vi "svfa_Modify Enhanced Spectrum Info (Dual).vi"(0 "spectrum info X":T3={"channel name"="", "description"="", "x-axis units"=0, "spectral info"={"spectrum type"=enum."Power [Magnitude^2]", "linear/dB"=enum."linear", "window"=0, "window size"=0, "FFT size"=0}, "engineering units"=0, "custom label"="", "dB reference [EU]"=0.0, "peak units"=enum."rms", "weighting filter"=0, "spectral density?"=FALSE, "unit label"="", "spectrum skewed?"=FALSE, "complimentary spectrum units"=enum."none"} {"x-axis units" items=["Time (s)"=0, "Frequency-CB (Hz)"=1, "Frequency-CPB (Hz)"=1248, "Frequency-Arbitrary (Hz)"=2357, "Quefrency (s)"=2, "Revolutions (rev)"=3, "Order"=4, "Speed (RPM)"=11, "Speed (rad/s)"=21, "Index"=65535]; "weighting filter" items=["Linear", "A-weighting", "B-weighting", "C-weighting", "ITU-R 468-4", "Dolby", "CCITT", "C-message", "Wb", "Wc", "Wd", "We", "Wf", "Wh", "Wj", "Wk", "Wm", "AES17 20 kHz lowpass", "AES17 40 kHz lowpass", "AES17 20 kHz highpass", "AES17 40 kHz highpass"]; "dB reference [EU]" format="%.2f"; "engineering units" items=["custom..."=0, "V"=1, "A"=21, "C"=30, "pC"=31, "s"=32, "-"=29, "Pa"=2, "N"=20, "g"=3, "m/s^2"=4, "m/s"=5, "m"=6, "mm/s"=12, "mm"=13, "micron/s"=14, "micron"=15, "in/s^2"=7, "in/s"=8, "in"=9, "mil/s"=10, "mil"=11, "rad/s^2"=16, "rad/s"=17, "rad"=18, "deg/s^2"=26, "deg/s"=27, "deg"=28, "RPM"=22, "cycle/s^2"=23, "Hz"=24, "cycle"=25, "strain"=19]; "spectral info"."window" items=["None "=0, "Hanning"=1, "Hamming"=2, "Blackman-Harris"=3, "Exact Blackman"=4, "Blackman"=5, "Flat Top"=6, "4 Term B-Harris "=7, "7 Term B-Harris"=8, "Low Sidelobe"=9, "Force - Exponential"=10, "Gaussian"=62]}, 1 "processing control":T1(ring), 5 "spectrum info Y":T3={"channel name"="", "description"="", "x-axis units"=0, "spectral info"={"spectrum type"=enum."Power [Magnitude^2]", "linear/dB"=enum."linear", "window"=0, "window size"=0, "FFT size"=0}, "engineering units"=0, "custom label"="", "dB reference [EU]"=0.0, "peak units"=enum."rms", "weighting filter"=0, "spectral density?"=FALSE, "unit label"="", "spectrum skewed?"=FALSE, "complimentary spectrum units"=enum."none"} {"x-axis units" items=["Time (s)"=0, "Frequency-CB (Hz)"=1, "Frequency-CPB (Hz)"=1248, "Frequency-Arbitrary (Hz)"=2357, "Quefrency (s)"=2, "Revolutions (rev)"=3, "Order"=4, "Speed (RPM)"=11, "Speed (rad/s)"=21, "Index"=65535]; "weighting filter" items=["Linear", "A-weighting", "B-weighting", "C-weighting", "ITU-R 468-4", "Dolby", "CCITT", "C-message", "Wb", "Wc", "Wd", "We", "Wf", "Wh", "Wj", "Wk", "Wm", "AES17 20 kHz lowpass", "AES17 40 kHz lowpass", "AES17 20 kHz highpass", "AES17 40 kHz highpass"]; "dB reference [EU]" format="%.2f"; "engineering units" items=["custom..."=0, "V"=1, "A"=21, "C"=30, "pC"=31, "s"=32, "-"=29, "Pa"=2, "N"=20, "g"=3, "m/s^2"=4, "m/s"=5, "m"=6, "mm/s"=12, "mm"=13, "micron/s"=14, "micron"=15, "in/s^2"=7, "in/s"=8, "in"=9, "mil/s"=10, "mil"=11, "rad/s^2"=16, "rad/s"=17, "rad"=18, "deg/s^2"=26, "deg/s"=27, "deg"=28, "RPM"=22, "cycle/s^2"=23, "Hz"=24, "cycle"=25, "strain"=19]; "spectral info"."window" items=["None "=0, "Hanning"=1, "Hamming"=2, "Blackman-Harris"=3, "Exact Blackman"=4, "Blackman"=5, "Flat Top"=6, "4 Term B-Harris "=7, "7 Term B-Harris"=8, "Low Sidelobe"=9, "Force - Exponential"=10, "Gaussian"=62]}, 11 "error in (no error)":errorcluster, 13 "spectrum type":T2) -> (3 "dup processing control":T1(ring), 4 "spectrum info":T3={"channel name"="", "description"="", "x-axis units"=0, "spectral info"={"spectrum type"=enum."Power [Magnitude^2]", "linear/dB"=enum."linear", "window"=0, "window size"=0, "FFT size"=0}, "engineering units"=0, "custom label"="", "dB reference [EU]"=0.0, "peak units"=enum."rms", "weighting filter"=0, "spectral density?"=FALSE, "unit label"="", "spectrum skewed?"=FALSE, "complimentary spectrum units"=enum."none"} {"x-axis units" items=["Time (s)"=0, "Frequency-CB (Hz)"=1, "Frequency-CPB (Hz)"=1248, "Frequency-Arbitrary (Hz)"=2357, "Quefrency (s)"=2, "Revolutions (rev)"=3, "Order"=4, "Speed (RPM)"=11, "Speed (rad/s)"=21, "Index"=65535]; "weighting filter" items=["Linear", "A-weighting", "B-weighting", "C-weighting", "ITU-R 468-4", "Dolby", "CCITT", "C-message", "Wb", "Wc", "Wd", "We", "Wf", "Wh", "Wj", "Wk", "Wm", "AES17 20 kHz lowpass", "AES17 40 kHz lowpass", "AES17 20 kHz highpass", "AES17 40 kHz highpass"]; "dB reference [EU]" format="%.2f"; "engineering units" items=["custom..."=0, "V"=1, "A"=21, "C"=30, "pC"=31, "s"=32, "-"=29, "Pa"=2, "N"=20, "g"=3, "m/s^2"=4, "m/s"=5, "m"=6, "mm/s"=12, "mm"=13, "micron/s"=14, "micron"=15, "in/s^2"=7, "in/s"=8, "in"=9, "mil/s"=10, "mil"=11, "rad/s^2"=16, "rad/s"=17, "rad"=18, "deg/s^2"=26, "deg/s"=27, "deg"=28, "RPM"=22, "cycle/s^2"=23, "Hz"=24, "cycle"=25, "strain"=19]; "spectral info"."window" items=["None "=0, "Hanning"=1, "Hamming"=2, "Blackman-Harris"=3, "Exact Blackman"=4, "Blackman"=5, "Flat Top"=6, "4 Term B-Harris "=7, "7 Term B-Harris"=8, "Low Sidelobe"=9, "Force - Exponential"=10, "Gaussian"=62]}, 15 "error out":errorcluster)   [LabVIEW 2017]
uses:
  <vilib>/addons/_NISVFA/_Shared subVIs/Controls/svc_Spectrum Info.ctl
  <vilib>/addons/_NISVFA/_Shared subVIs/Controls/svc_X-Axis Units.ctl
  <vilib>/addons/_NISVFA/_Shared subVIs/Controls/svc_Spectrum Type.ctl
  <vilib>/addons/_NISVFA/_Shared subVIs/Controls/svc_Engineering Units Text Ring.ctl
  <vilib>/addons/_NISVFA/_Shared subVIs/Controls/svc_Weighting Filter Text Ring.ctl
  <vilib>/addons/_NISVFA/_Shared subVIs/Controls/svc_Complimentary Spectrum Units.ctl
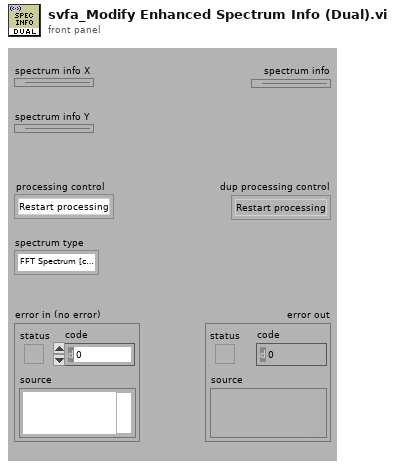
[diagram p1: front panel]
types:
  T1 = enum16{"Restart processing", "Continue processing", "Skip processing"}
  T2 = typedef "svc_Spectrum Type.ctl" = enum16{"FFT Spectrum [complex]", "Amplitude [Magnitude]", "Power [Magnitude^2]", "Cross Spectrum [complex]", "Frequency Response [Complex]"}
  T3 = typedef "svc_Spectrum Info.ctl" = cluster{"channel name":string, "description":string, "x-axis units":T4, "spectral info":cluster{"spectrum type":T2, "linear/dB":enum16{"linear", "dB"}, "window":u16, "window size":i32, "FFT size":i32}, "engineering units":T5, "custom label":string, "dB reference [EU]":dbl, "peak units":enum16{"rms", "peak", "peak-peak"}, "weighting filter":T6, "spectral density?":bool, "unit label":string, "spectrum skewed?":bool, "complimentary spectrum units":T7}
  T4 = typedef "svc_X-Axis Units.ctl" = u16
  T5 = typedef "svc_Engineering Units Text Ring.ctl" = u16
  T6 = typedef "svc_Weighting Filter Text Ring.ctl" = u16
  T7 = typedef "svc_Complimentary Spectrum Units.ctl" = enum16{"none", "radians", "degrees", "cycles", "imaginary"}
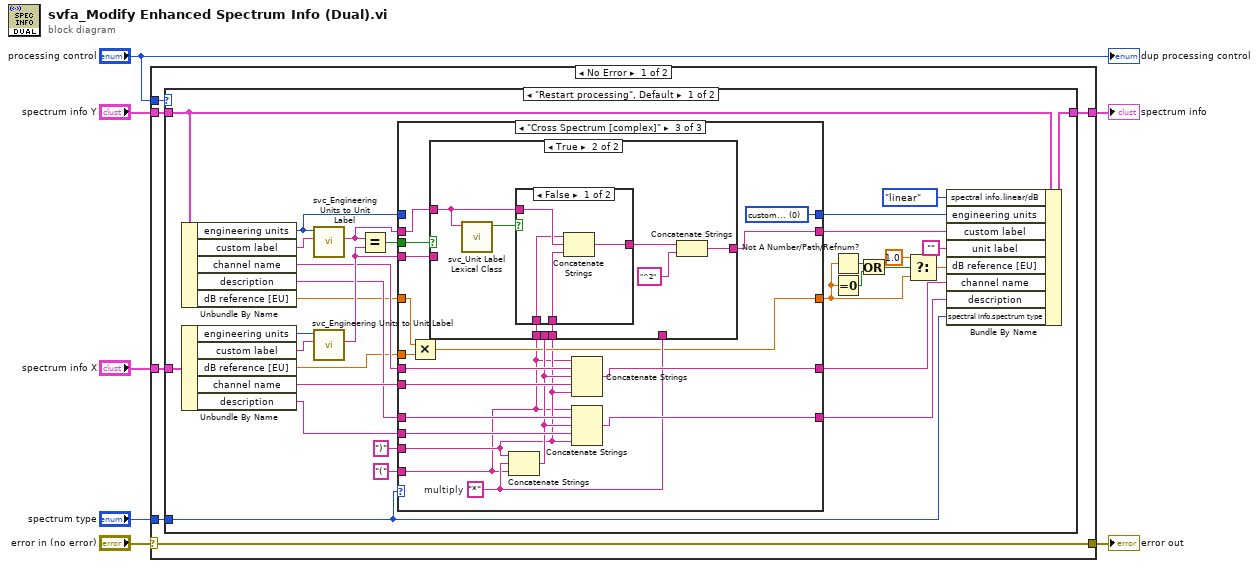
[diagram p0: block diagram]
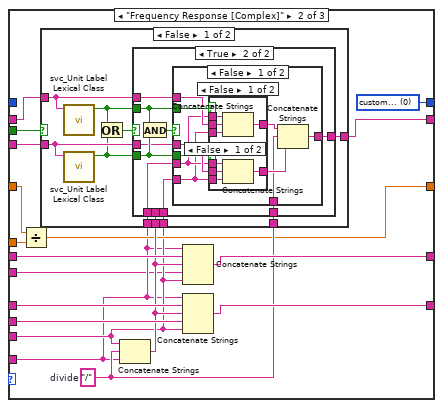
[diagram p3: hidden frame]
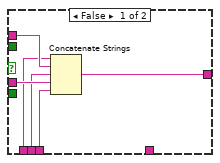
[diagram p4: hidden frame]
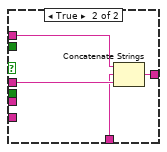
[diagram p7: hidden frame]
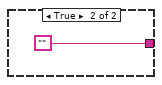
[diagram p8: hidden frame]
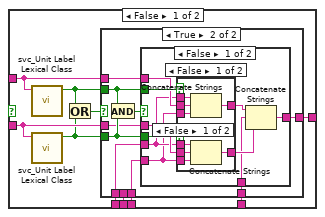
[diagram p9: hidden frame]
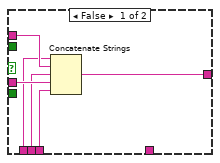
[diagram p10: hidden frame]
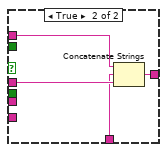
[diagram p13: hidden frame]
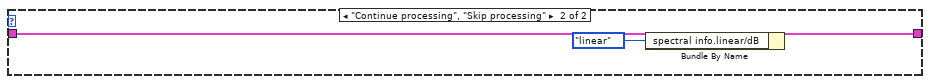
[diagram p15: hidden frame]
diagram:
  n1 = case shown="No Error" "error in (no error)" {
    selector: "error in (no error)" -> [w10 w201]
    tunnel: [w8 w200] -> w7
    tunnel: [w10 w201] -> w5
    tunnel: "spectrum type" -> [w13 _]
    tunnel: "spectrum info Y" -> [w12 w200]
    tunnel: "spectrum info X" -> [w11 _]
    tunnel: "processing control" -> [w9 _]
    frame No Error {
      n2 = case shown="\"Restart processing\", Default" w9 {
        tunnel: [w44 w198] -> w8
        tunnel: w13 -> [w22 _]
        tunnel: w12 -> [w43 w199]
        tunnel: w11 -> [w42 _]
        frame "Restart processing", Default {
          n3 = Unbundle By Name(w43) -> ("engineering units"=w18:T5, "custom label"=w26:string, "channel name"=w25:string, "description"=w24:string, "dB reference [EU]"=w23:dbl)
          n4 = Unbundle By Name(w42) -> ("engineering units"=w30:T5, "custom label"=w29:string, "dB reference [EU]"=w19:dbl, "channel name"=w33:string, "description"=w32:string)
          n5 = call <vilib>:"svc_Engineering Units to Unit Label.vi"("custom label"=w26, "engineering units"=w18) -> ("unit label"=w27:string)  [unwired: 8 in, 1 out]
          n6 = call <vilib>:"svc_Engineering Units to Unit Label.vi"("custom label"=w29, "engineering units"=w30) -> ("unit label"=w28:string)  [unwired: 8 in, 1 out]
          n7 = Equal?(x=w27, y=w28) -> (x = y?=w31:bool)
          n8 = case shown="\"Cross Spectrum [complex]\"" w22 {
            tunnel: [w46 w53 w120] -> w36
            tunnel: w31 -> [_ w67 w135]
            tunnel: w27 -> [w45 w66 w134]
            tunnel: [w45 w65 w133] -> w14
            tunnel: w28 -> [_ w64 w132]
            tunnel: [w47 w63 w131] -> w17
            tunnel: w33 -> [_ w50 w129]
            tunnel: w25 -> [w49 w62 w130]
            tunnel: [w49 w61 w128] -> w34
            tunnel: w32 -> [_ w59 w126]
            tunnel: w24 -> [w48 w60 w127]
            tunnel: [w48 w58 w125] -> w35
            tunnel: w18 -> [w47 _ _]
            tunnel: w23 -> [w46 w54 w123]
            tunnel: w19 -> [_ w55 w122]
            tunnel: ")" ("Substring") -> [_ w52 w119]
            tunnel: "(" ("Substring") -> [_ w51 w118]
            frame "Power [Magnitude^2]", Default {
            }
            frame "Frequency Response [Complex]" {
              w56 = "/"  # divide
              w63 = T5 0 items=["custom..."=0, "V"=1, "A"=21, "Pa"=2, "N"=20, "g"=3, "m/s^2"=4, "m/s"=5, "m"=6, "mm/s"=12, "mm"=13, "microns/s"=14, "microns"=15, "in/s^2"=7, "in/s"=8, "in"=9, "mils/s"=10, "mils"=11, "rad/s^2"=16, "rad/s"=17, "rad"=18, "strain"=19] ("engineering units")
              n9 = Divide(x=w54, y=w55) -> (x/y=w53:dbl)
              n10 = Concatenate Strings(w52, w56, w51) -> (w57:string)
              n11 = case shown="False" w67 {
                tunnel: w66 -> [w73 _]
                tunnel: [w77 "" ("Empty String Constant")] -> w65
                tunnel: w64 -> [w72 _]
                tunnel: w52 -> [w76 _]
                tunnel: w57 -> [w75 _]
                tunnel: w51 -> [w74 _]
                tunnel: w56 -> [w68 _]
                frame False {
                  n12 = call <vilib>:"svc_Unit Label Lexical Class.vi"("unit label"=w73) -> ("letters only?"=w70:bool)  [unwired: 6 in]
                  n13 = call <vilib>:"svc_Unit Label Lexical Class.vi"("unit label"=w72) -> ("letters only?"=w69:bool)  [unwired: 6 in]
                  n14 = Or(x=w70, y=w69) -> (x .or. y?=w71:bool)
                  n15 = case shown="True" w71 {
                    tunnel: w73 -> [w83 w89]
                    tunnel: w72 -> [w82 w88]
                    tunnel: [w81 w87] -> w77
                    tunnel: w76 -> [w80 w85]
                    tunnel: w75 -> [w79 _]
                    tunnel: w74 -> [w78 w86]
                    tunnel: w70 -> [_ w91]
                    tunnel: w69 -> [_ w92]
                    tunnel: w68 -> [_ w84]
                    frame False {
                      n16 = Concatenate Strings(w78, w83, w79, w82, w80) -> (w81:string)
                    }
                    frame True {
                      n17 = And(x=w91, y=w92) -> (x .and. y?=w90:bool)
                      n18 = case shown="False" w90 {
                        tunnel: w92 -> [w99 _]
                        tunnel: w91 -> [w102 _]
                        tunnel: w89 -> [w101 w116]
                        tunnel: w88 -> [w100 w115]
                        tunnel: [w94 w114] -> w87
                        tunnel: w86 -> [w98 _]
                        tunnel: w85 -> [w97 _]
                        tunnel: w84 -> [w93 w113]
                        frame False {
                          n19 = case shown="False" w102 {
                            tunnel: w101 -> [w111 w112]
                            tunnel: [w108 w112] -> w96
                            tunnel: w98 -> [w110 _]
                            tunnel: w97 -> [w109 _]
                            frame False {
                              n20 = Concatenate Strings(w110, w111, w109) -> (w108:string)
                            }
                            frame True {
                            }
                          }
                          n21 = case shown="False" w99 {
                            tunnel: w100 -> [w106 w107]
                            tunnel: [w105 w107] -> w95
                            tunnel: w98 -> [w104 _]
                            tunnel: w97 -> [w103 _]
                            frame False {
                              n22 = Concatenate Strings(w104, w106, w103) -> (w105:string)
                            }
                            frame True {
                            }
                          }
                          n23 = Concatenate Strings(w96, w93, w95) -> (w94:string)
                        }
                        frame True {
                          n24 = Concatenate Strings(w116, w113, w115) -> (w114:string)
                        }
                      }
                    }
                  }
                }
                frame True {
                }
              }
              n25 = Concatenate Strings(w51, w62, w57, w50, w52) -> (w61:string)
              n26 = Concatenate Strings(w51, w60, w57, w59, w52) -> (w58:string)
            }
            frame "Cross Spectrum [complex]" {
              w121 = "*"  # multiply
              w131 = T5 0 items=["custom..."=0, "V"=1, "A"=21, "Pa"=2, "N"=20, "g"=3, "m/s^2"=4, "m/s"=5, "m"=6, "mm/s"=12, "mm"=13, "microns/s"=14, "microns"=15, "in/s^2"=7, "in/s"=8, "in"=9, "mils/s"=10, "mils"=11, "rad/s^2"=16, "rad/s"=17, "rad"=18, "strain"=19] ("engineering units")
              n27 = Multiply(x=w123, y=w122) -> (x*y=w120:dbl)
              n28 = Concatenate Strings(w119, w121, w118) -> (w124:string)
              n29 = case shown="True" w135 {
                tunnel: w134 -> [w141 w188]
                tunnel: [w145 w185] -> w133
                tunnel: w132 -> [w140 _]
                tunnel: w119 -> [w144 w186]
                tunnel: w124 -> [w143 _]
                tunnel: w118 -> [w142 w187]
                tunnel: w121 -> [w136 _]
                frame False {
                  n30 = call <vilib>:"svc_Unit Label Lexical Class.vi"("unit label"=w141) -> ("letters only?"=w138:bool)  [unwired: 6 in]
                  n31 = call <vilib>:"svc_Unit Label Lexical Class.vi"("unit label"=w140) -> ("letters only?"=w137:bool)  [unwired: 6 in]
                  n32 = Or(x=w138, y=w137) -> (x .or. y?=w139:bool)
                  n33 = case shown="True" w139 {
                    tunnel: w141 -> [w151 w157]
                    tunnel: w140 -> [w150 w156]
                    tunnel: [w149 w155] -> w145
                    tunnel: w144 -> [w148 w153]
                    tunnel: w143 -> [w147 _]
                    tunnel: w142 -> [w146 w154]
                    tunnel: w138 -> [_ w159]
                    tunnel: w137 -> [_ w160]
                    tunnel: w136 -> [_ w152]
                    frame False {
                      n34 = Concatenate Strings(w146, w151, w147, w150, w148) -> (w149:string)
                    }
                    frame True {
                      n35 = And(x=w159, y=w160) -> (x .and. y?=w158:bool)
                      n36 = case shown="False" w158 {
                        tunnel: w160 -> [w167 _]
                        tunnel: w159 -> [w170 _]
                        tunnel: w157 -> [w169 w184]
                        tunnel: w156 -> [w168 w183]
                        tunnel: [w162 w182] -> w155
                        tunnel: w154 -> [w166 _]
                        tunnel: w153 -> [w165 _]
                        tunnel: w152 -> [w161 w181]
                        frame False {
                          n37 = case shown="False" w170 {
                            tunnel: w169 -> [w179 w180]
                            tunnel: [w176 w180] -> w164
                            tunnel: w166 -> [w178 _]
                            tunnel: w165 -> [w177 _]
                            frame False {
                              n38 = Concatenate Strings(w178, w179, w177) -> (w176:string)
                            }
                            frame True {
                            }
                          }
                          n39 = case shown="False" w167 {
                            tunnel: w168 -> [w174 w175]
                            tunnel: [w173 w175] -> w163
                            tunnel: w166 -> [w172 _]
                            tunnel: w165 -> [w171 _]
                            frame False {
                              n40 = Concatenate Strings(w172, w174, w171) -> (w173:string)
                            }
                            frame True {
                            }
                          }
                          n41 = Concatenate Strings(w164, w161, w163) -> (w162:string)
                        }
                        frame True {
                          n42 = Concatenate Strings(w184, w181, w183) -> (w182:string)
                        }
                      }
                    }
                  }
                }
                frame True {
                  n43 = call <vilib>:"svc_Unit Label Lexical Class.vi"("unit label"=w188) -> ("letters only?"=w191:bool)  [unwired: 6 in]
                  n44 = case shown="False" w191 {
                    tunnel: [w194 w196] -> w189
                    tunnel: w188 -> [w195 w196]
                    tunnel: w187 -> [w193 _]
                    tunnel: w186 -> [w192 _]
                    frame False {
                      n45 = Concatenate Strings(w193, w195, w192) -> (w194:string)
                    }
                    frame True {
                    }
                  }
                  n46 = Concatenate Strings(w189, "^2" ("Substring")) -> (w185:string)
                }
              }
              n47 = Concatenate Strings(w118, w130, w124, w129, w119) -> (w128:string)
              n48 = Concatenate Strings(w118, w127, w124, w126, w119) -> (w125:string)
            }
          }
          n49 = Not A Number/Path/Refnum?(number/path/refnum=w36) -> (NaN/Path/Refnum?=w41:bool)
          n50 = Equal To 0?(x=w36) -> (x = 0?=w37:bool)
          n51 = Or(x=w41, y=w37) -> (x .or. y?=w40:bool)
          n52 = Select(t=1.0, s=w40, f=w36) -> (s? t:f=w38:dbl)
          n53 = Bundle By Name(cluster=w43, "spectral info.linear/dB"=enum16{"linear", "dB"}."linear", "engineering units"=w17, "custom label"=w14, "unit label"="" ("Empty String Constant"), "dB reference [EU]"=w38, "channel name"=w34, "description"=w35, "spectral info.spectrum type"=w22) -> (w44:T3)
        }
        frame "Continue processing", "Skip processing" {
          n54 = Bundle By Name(cluster=w199, "spectral info.linear/dB"=enum16{"linear", "dB"}."linear") -> (w198:T3)
        }
      }
    }
    frame Error {
    }
  }
  "spectrum info" <- w7
  "error out" <- w5
  "dup processing control" <- "processing control"
